vi "Generate Support files File paths.vi"(4 "error in":errorcluster, 6 "base path":path, 7 "ProjectName":T1) -> (0 "error out":errorcluster, 1 "Log path":path, 2 ".ini path":path)   [LabVIEW 2013]
doc: "This .vi generates the filepaths to the various support files and stores that in a global."
uses:
  Config/ProjectName enum.ctl
  Config/User interface config file selector enum.ctl
  Config/Config file functional global mode enum.ctl
  FileIO lib.lvlib
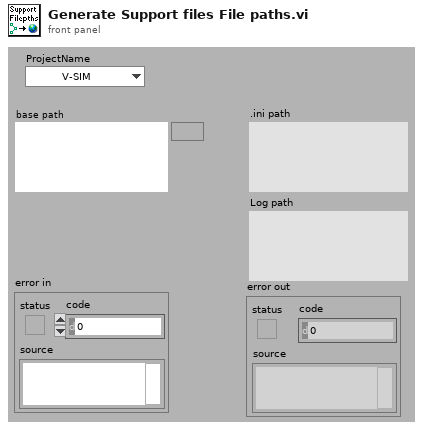
[diagram p1: front panel]
types:
  T1 = typedef "ProjectName enum.ctl" = enum16{"V-SIM", "SPIM", "TEMca2", "undefined", "HHMI Panels"}
  T2 = typedef "User interface config file selector enum.ctl" = enum16{"MAIN"}
  T3 = typedef "Config file functional global mode enum.ctl" = enum16{"Set Filepath", "Read file", "Rewrite file"}
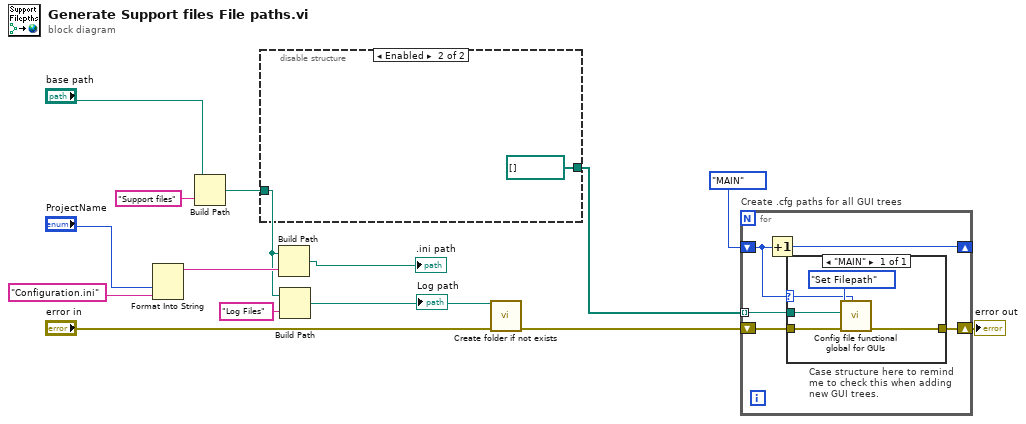
[diagram p0: block diagram]
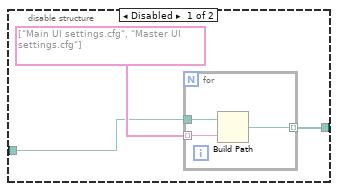
[diagram p2: hidden frame]
diagram:
  n1 = Format Into String("ProjectName", "Configuration.ini" ("name or relative path")) -> (resulting string=w11:string)  [unwired: 3 in, 1 out]
  n2 = Build Path(base path="base path", name or relative path="Support files" ("string")) -> (appended path=w6:path)
  n3 = disable-structure shown="Enabled" {
    disable-tunnel: [w17 path[] []] -> w4
    disable-tunnel: w6 -> [w15 _]
    frame Disabled {
      n4 = for {
        tunnel: w15 -> [w20]
        tunnel: [w19] -> w17 mode=indexing
        tunnel: string[] ["Main UI settings.cfg", "Master UI settings.cfg"] -> [w18] mode=indexing
        n5 = Build Path(base path=w20, name or relative path=w18) -> (appended path=w19:path)
      }
    }
    frame Enabled {
    }
  }
  n6 = Build Path(base path=w6, name or relative path=w11) -> (appended path=→".ini path":path)
  n7 = Build Path(base path=w6, name or relative path="Log Files") -> (appended path=w3:path)
  "Log path" <- w3
  n8 = call "Create folder if not exists.vi"("error in"="error in", "Path in"=w3) -> ("error out"=w1:errorcluster)  [unwired: 7 in, 2 out]
  n9 = for "Create .cfg paths for all GUI trees" {
    tunnel: w4 -> [w25] mode=indexing
    shift-right: [w24] -> w14
    shift-left: w1 -> [w26]
    shift-right: [w23] -> _
    shift-left: User_interface_config_file_selector_enum."MAIN" ("Config file") -> [w22]
    # "Case structure here to remind\nme to check this when adding\nnew GUI trees."
    n10 = Increment(x=w22) -> (x+1=w23:T2)
    n11 = case shown="\"MAIN\"" w22 {
      selector: w22 -> [w27]
      tunnel: w26 -> [w30]
      tunnel: w25 -> [w29]
      tunnel: [w28] -> w24
      frame "MAIN" {
        n12 = call "Config file functional global for GUIs.vi"("GUI elements"=w27, "error in"=w30, "file path"=w29, "Mode"=Config_file_functional_global_mode_enum."Set Filepath") -> ("error out"=w28:errorcluster)  [unwired: 1 in, 6 out]
      }
    }
  }
  "error out" <- w14
